vi "AlliGator All ROIs Decay Fit.vi"(8 "error in (no error)":errorcluster, 10 "Lifetime Graph":refnum<vi>, 11 "AlliGator Internal Variables DVR":refnum<data-value>) -> (0 "error out":errorcluster, 1 "Message":string, 3 "AlliGator Internal Variables DVR":refnum<data-value>)   [LabVIEW 2021, in "AlliGator Decay Fit.lvlib"]
doc: "Fits all ROI decays with the selected model, using a common IRF for all ROIs."
uses:
  AlliGator Decay Fit.lvlib
  Internal Variables/AlliGator Internal Variables v2.ctl
  <vilib>/vision/Image Controls.llb/IMAQ Image.ctl
  Internal Variables/AlliGator Gate Image Set.ctl
  Files/AlliGator FLI Dataset Type.ctl
  Files/AlliGator Data Series Type.ctl
  Dual-Channel Datasets/AlliGator Dataset Channel.ctl
  Settings/AlliGator Gate Arithmetic.ctl
  Source Image/AlliGator Displayed Image.ctl
  Image/Named ROI Description.ctl
  Phasor Graph/AlliGator Decay Metadata v3.ctl
  Decay Preprocessing/AlliGator Decay Background Subtraction Info.ctl
  Decay Preprocessing/AlliGator Baseline Subtraction Method.ctl
  Graphs/XY Graph/XY Graph Plot Shift Parameters.ctl
  Graphs/XY Graph/XY Graph Plot Shift Method.ctl
  Decay Preprocessing/AlliGator Decay Extrapolation Parameters.ctl
  Phasor/Calibration Phasor (m, phi).ctl
  Phasor/Phasor Reference Series.ctl
  Phasor/Phasor Calibration Map v2.ctl
  Phasor/Phasor (g, s).ctl
  Phasor Graph/AlliGator Raw Phasor Plot Data v5.ctl
  Phasor/Phasor Standard Deviation Options.ctl
  Phasor Plot/AlliGator Phasor Multi-Harmonic Data.ctl
  Phasor/Phasor Harmonic Data.ctl
  Decay Fit Parameter Map/AlliGator Decay Fit Options & Parameters v4.ctl
  Fits/IRF(X)PSED/Decay Fit Options v4.ctl
  Fits/Decay Convolution/Decay Model.ctl
  Fits/Residual Type.ctl
  Fits/IRF(X)PSED/Fit Weights Type v2.ctl
  Fits/Non-linear Fitting Method v2.ctl
  Fits/Fit Calculation Method.ctl
  Fits/Non-linear Fitting Algorithm.ctl
  AlliGator Decay Fit Parameter Constraints 2.ctl
  Fits/IRF(X)PSED/Decay Fit Parameters In List.ctl
  Fits/IRF(X)PSED/MLE Baseline Offset Type.ctl
  Decay Preprocessing/AlliGator Decay Preprocessing Parameters.ctl
  Fits/IRF(X)PSED/Decay Fit Parameters & Derived Quantities List v2.ctl
  Fits/IRF(X)PSED/Decay Fit Result Constraint.ctl
  Decay Fit Parameter Map/AlliGator Parameter Maps Data.ctl
  Globals, Variables, Constants/AlliGator Variables List.ctl
  Settings/AlliGator Settings List.ctl
  Rich Text Box/Text Format List.ctl
  Graphs/XY Graph/XY Graph Selected Plot Info+Flag.ctl
  Graphs/XY Graph/XY Graph Refnum.ctl
  <vilib>/Utility/miscctls.llb/LVPoint32TypeDef.ctl
  Variant/Variant to Data/Variant to U16.vi
  Variant/Variant to Data/Variant to Boolean.vi
  Globals, Variables, Constants/AlliGator Abort.vi
  <vilib>/Utility/error.llb/Error Cluster From Error Code.vi
  <vilib>/ErrorRing/Error Ring.xnode
  Globals, Variables, Constants/AlliGator Globals, Variables & Constants.lvlib
  Image/Image.lvlib
  Decay Processing/AlliGator Decay Processing.lvlib
  Source Image/AlliGator Source Image.lvlib
  Strings/Strings.lvlib
  Time/Time.lvlib
  Graphs/XY Graph/XY Graph Add-Ons.lvlib
  Settings/AlliGator Settings.lvlib
  Decay Preprocessing/AlliGator Decay Preprocessing.lvlib
  Fits/Fits.lvlib
  Variant/Variant to Data/Variant to Data.lvlib
  Notebook/Notebook.lvlib
  GUI/GUI.lvlib
  Utilities/Utilities.lvlib
  Error/Error.lvlib
  Decay Fit Parameter Map/AlliGator Decay Fit Parameter Map.lvlib
  Phasor/Phasor.lvlib
  Files/AlliGator Files.lvlib
  Internal Variables/AlliGator Internal Variables.lvlib
  Phasor Graph/AlliGator Phasor Graph.lvlib
  Phasor Plot/AlliGator Phasor Plot.lvlib
  Dual-Channel Datasets/AlliGator Dual-Channel Datasets.lvlib
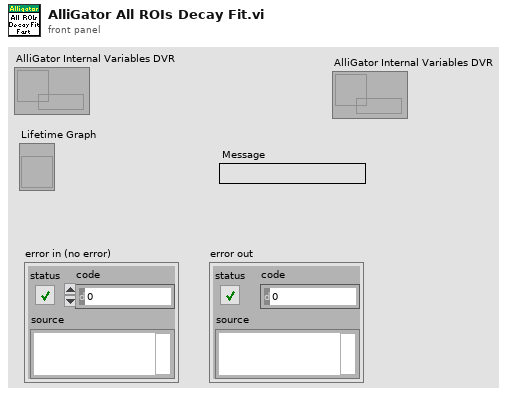
[diagram p1: front panel]
types:
  T1 = typedef "AlliGator Decay Fit.lvlib/AlliGator Decay Fit Output Options.ctl" = cluster{"Fit Model":T2, "Decay Fit Parameter Array":T3[]}
  T2 = typedef "Fits.lvlib/Decay Model.ctl" = enum16{"1-Exponential", "2-Exponentials"}
  T3 = typedef "Fits.lvlib/Decay Fit Parameters & Derived Quantities List v2.ctl" = enum16{"Offset", "Baseline", "A_1", "tau_1", "A_2", "tau_2", "<tau>_a", "f1_a", "f2_a", "<tau>_i", "f1_i", "f2_i", "-", "R^2", "Chi^2"}
  T4 = typedef "AlliGator Globals, Variables & Constants.lvlib/AlliGator Variables List.ctl" = enum16{"---- GUI ----", "GUI:Initialization Status", "GUI:State Indicators Refnum", "GUI:Original AlliGator Menu Items", "GUI:Current Action Loop State", "GUI:Script in progress", "GUI:Playback", "GUI:Loop Playback", "GUI:Search ROI Used", "GUI:Search ROI", "Decay Graph Max Legend Size", "Intensity Graph Max Legend Size", "Decay Statistics Graph Max Legend Size", "Phasor Graph Max Legend Size", "Phasor Ratio Graph Max Legend Size", "Lifetime Graph Max Legend Size", "---- Files ----", "Files:Export Dataset Frames as Individual Files", "Files:Show Batch Export Help Balloons", "Files:Frames in Dataset", "Files:ptu File Frame Start Indices", "Files:Current Frame in Dataset", "Files:Current Frame Timestamp", "Files:Dataset Loaded", "Files:Dataset Metadata", "Files:Dataset Channel", "Files:Dataset Data Description", "Files:Background Dataset Metadata", "Files:Background Dataset Channel", "Files:Background Dataset Data Description", "Files:Background File Subtraction", "Files:Background File Path", "Files:Background File Pile-up Correction", "Files:Background File Pixel Well Capacity", "Files:Background File Scaling Factor", "Files:Current Dataset Load Settings", "Files:Dataset Path", "Files:ICCD-specific Information", "Files:Macrotime Gate Separation", "------ Python Plugins ------", "Python Plugins:Information", "Python Plugins:Python Session", "Python Plugins:Valid Python Session?", "---- Source Image ----", "Source Image:ROIs", "Source Image:Current ROI", "Source Image:ROI Event Refnum", "X_Source Image:Display Range", "X_Source Image:Palette Information", "X_Source Image:Type of Displayed Image", "X_Time Gate Slider", "Source Image:Palette List", "Source Image:Scale", "Source Image:ROI Overlay Color", "Source Image:Overlay to Erase", "Source Image:Is Displayed Image Accumulated", "Source Image:White Light Image Modified", "Source Image:Mask Image Modified", "---- Image Profile Window ----", "Image Profile:Window Event Refnum", "Image Profile:IntensityType", "Image Profile:Intensity Average Type", "Image Profile:Intensity-weighted SDV", "Image Profile:Box Profile Type", "Image Profile:Window Open", "Image Profile:Plotted Fit Parameter", "------ Phasor Graph -------", "Phasor Graph:Show Line", "---- Phasor Plot ---", "Phasor Plot:Parameters Changed", "Phasor Plot:FLI Dataset Modified since last Calculation", "Phasor Harmonics Data", "Selected Phasor Harmonics", "Phasor Harmonic Manager Event Refnum", "Phasor Plot:ROIs", "Phasor Plot:Current ROI", "Phasor Plot:ROI Event Refnum", "Phasor Plot:Image Reference Points", "Phasor Plot:Computed", "Phasor Plot:Palette Information", "Phasor Plot:Palette List", "Phasor Plot:Phasor Ratio Palette Information", "Phasor Plot:Phasor Ratio Palette List", "Phasor Plot:Image Scale", "Phasor Plot:Image Overlay to Erase", "Phasor Plot:Image Elements to Update", "Phasor Plot:Current Calculation Parameters", "Phasor Plot:Current Calibration Options", "Phasor Plot:Reset Cumulated Phasor Plot", "Phasor Plot:Reference 1", "Phasor Plot:Lifetime Reference 1", "Phasor Plot:Reference 1 Frequency", "Phasor Plot:Reference 2", "Phasor Plot:Lifetime Reference 2", "Phasor Plot:Reference 2 Frequency", "---- Decay Analysis ----", "Number of Selected Decays to Fit", "LS Fit Results", "LAR Fit Results", "BS Fit Results", "Last Decay Max - Min", "Best Fit Parameters", "Best Fit Parameter Names", "Actual Size X", "Actual Size Y", "Binning X", "Binning Y", "Actual # Gates", "Dataset Number", "Gates to...", "Gates Skipped", "Gates to keep", "Gate Step", "Gate Separation", "Reversed Gates", "Pile-up Correction", "Pixel Well Capacity", "Background Subtracted", "Background Subtraction Method", "Background Definition Range", "Background File (deprecated)", "Number of Dataset Accumulated", "Array of Accumulated Dataset Paths", "Do Averaged Datasets", "Destination File Path", "Process Plot Target", "Use 1/D as Phasor Frequency", "---- Decay Fit Parameter Map -----", "Decay Fit Parameter Map:Palette Information", "Decay Fit Parameter Map:Palette List", "Decay Fit Parameter Map:X Resolution", "Decay Fit Parameter Map:Y Resolution", "Decay Fit Parameter Map:Use Decay Fit Result Constraints", "Decay Fit Parameter Map:Decay Fit Result Constraints", "Decay Fit Parameter Map:Decay Fit Result Constraints Applied", "---- Parameter Map ----", "Parameter Map:Palette Information", "Parameter Map:Palette List", "------- Local Decay Window ---------", "Local Decay Graph Window:Event Refnum", "Local Decay Graph Window:Use normalized IRF for convolution", "----- Miscellaneous ----", "Misc:Skippable Dialog Windows Status"}
  T5 = typedef "IMAQ Image.ctl" = refnum<image>
  T6 = typedef "AlliGator Settings.lvlib/AlliGator Settings List.ctl" = enum16{"GUI:Visible Settings Tab", "GUI:Last Run Version", "Source Image:Use Image Histogram for Contrast", "Source Image:Low Count Pixels Rejection Options", "Source Image:High Count Pixels Rejection Options", "Source Image:Use Image Brightness", "Source Image:Blend Overlay with Image Background", "Source Image:Use Fixed ROI Diameter", "Source Image:ROI Diameter", "Source Image:ROI Center Color", "Source Image:Peak Threshold", "Source Image:Intensity Threshold", "Source Image:Image Binning Options", "Source Image:Image Smoothing Options", "Source Image:Image Histogram Active", "Source Image:Invert Binary Mask", "Source Image:Hot Pixel Removal", "Source Image:Overlay Analyzed ROI Center", "Source Image:Auto-Adjust Contrast", "Source Image:Histogram Lower Percentile", "Source Image:Histogram Upper Percentile", "Source Image:Save Source Image", "Source Image:Scale Bar Options", "Source Image:Image Resolution (Pixel Size)", "Source Image:Flatfield Correction", "Source Image:Show Dead Left Columns Correction", "Source Image:Dead Left Columns Correction", "Source Image:Image Pre-Processing Operations Order", "Source Image:Overlay ROI Median", "Source Image:Median Overlay Color", "Data Information:Gate Width", "Data Information:Nanotime Gate Separation", "Data Information:Macrotime Gate Separation", "Data Information:Gate Step", "Data Information:# Gates", "Data Information:Gate Image Exposure", "Data Information:Gate Image Integration", "Data Information:Gates to Skip", "Data Information:Gates to Keep", "Data Information:Define Gates to", "Data Information:Channel Name", "Data Information:Available Channel Names", "Data Information:Channel Arithmetic", "Data Information:Background File Subtraction", "Data Information:Background File", "Data Information:Background Scaling Factor", "Data Information:Background Pile-up Correction", "Data Information:Background Pixel Well Capacity", "Data Information:Laser Period", "Data Information:SYNC Period", "Data Information:Pile-up Correction", "Data Information:Pixel Well Capacity", "Data Information:Dataset Scaling Factor", "Fluorescence Decay_Decay Pre-Processing:Reverse Gates", "Fluorescence Decay_Decay Pre-Processing:Verbose Decay Pre-Processing", "Fluorescence Decay_Decay Pre-Processing:Use Decay Pre-Processing", "Fluorescence Decay_Decay Pre-Processing:Background Subtraction", "Fluorescence Decay_Decay Pre-Processing:Background Definition Range", "Fluorescence Decay_Decay Pre-Processing:Baseline Subtraction Method", "Fluorescence Decay_Decay Pre-Processing:Decay Pre-Processing Operations Order", "Fluorescence Decay_Decay Pre-Processing:Smoothing Parameter", "Fluorescence Decay_Decay Pre-Processing:Shift Decay", "Fluorescence Decay_Decay Pre-Processing:Decay Shift Parameters", "Fluorescence Decay_Decay Pre-Processing:Fold Decay", "Fluorescence Decay_Decay Pre-Processing:# Folds", "Fluorescence Decay_Decay Pre-Processing:1-Normalize Decay", "Fluorescence Decay_Decay Pre-Processing:[0-1]-Normalize Decay", "Fluorescence Decay_Decay Pre-Processing:Smoothen Decay", "Fluorescence Decay_Decay Pre-Processing:Extrapolate Decay", "Fluorescence Decay_Decay Pre-Processing:Use Periodicity", "Fluorescence Decay_Decay Pre-Processing:Use Cursors", "Fluorescence Decay_Decay Pre-Processing:Tail Fraction", "Fluorescence Decay_Decay Pre-Processing:Head Fraction", "Fluorescence Decay_Decay Pre-Processing:Additional Points", "Fluorescence Decay_Decay Pre-Processing:Straighten Decay", "Fluorescence Decay_Decay Pre-Processing:Constant Background", "Fluorescence Decay_Decay Pre-Processing:Pixel-Normalize Decay", "Fluorescence Decay_Advanced Analysis:Extract IRF instead of Decay", "Fluorescence Decay_Advanced Analysis:IRF Extraction Options", "Fluorescence Decay_Advanced Analysis:IRF Optimization Options", "Fluorescence Decay_Advanced Analysis:Square Pulse Options", "Fluorescence Decay_Advanced Analysis:IRF Order", "Fluorescence Decay_Advanced Analysis:IRF Time Constants", "Fluorescence Decay_Advanced Analysis:Wavelet Analysis Options", "Fluorescence Decay_Advanced Analysis:Average Lifetime Options", "Fluorescence Decay_Fit Options:Fit Options", "Fluorescence Decay_Fit Options:Use Legacy Fitting Approach", "Fluorescence Decay_Fit Options:Use Data Information Laser Period", "Fluorescence Decay_Fit Parameters:Displayed Fit Parameters", "Fluorescence Decay_Fit Parameters:Fit Parameter Constraints", "Fluorescence Decay_Fit Parameters:Export Tabulated Results", "Fluorescence Decay_Fit Parameters:MLE Baseline Offset Type", "Fluorescence Decay_Fit Parameters:MLE Baseline Offset", "Fluorescence Decay_Fit Parameters:Guess Parameter Names", "Fluorescence Decay_Fit Parameters:Guess Parameter Values", "Fluorescence Decay_Fit Parameters:Guess Parameters Options", "Fluorescence Decay_Fit Parameters:Optimal Offset Selection Criterion", "Fluorescence Decay_Styles:Show Last Decay Only", "Fluorescence Decay_Styles:Decay Graph Color Array", "Fluorescence Decay:Decay Graph Active", "Fluorescence Decay Statistics:Min Peak Value", "Fluorescence Decay Statistics:Reject Low Decay Peak Pixels", "Fluorescence Decay Statistics:Reject High Decay Peak Pixels", "Fluorescence Decay Statistics:Max Peak Value", "Time Traces:Use File Timestamp", "Time Traces:Time Step", "Time Traces:Use Intensity Correction File", "Time Traces:Intensity Correction File", "Phasor Plot:Phasor Plot Smoothing Options", "Phasor Plot:Phasor Plot Size", "Phasor Plot:Phasor Plot Graphics Options", "Phasor Plot:Cumulative Phasor Plot", "Phasor Plot:Use Phasor Brightness", "Phasor Plot:Blend Overlay with Phasor Background", "Phasor Plot:Save Phasor Plot", "Phasor Plot:Show References", "Phasor Plot:Phasor Ratio Decay Range", "Phasor Plot:Exponential Fading", "Phasor Plot:Phasor Ratio Reference Colors", "Phasor Plot:Reference Radius", "Phasor Plot:Show Color Map Vertices", "Phasor Plot:Phasor Plot Active", "Phasor Plot:Phasor Ratio Color Map Type", "Phasor Plot:Phasor Ratio Color Map", "Phasor Plot:Phasor Ratio Display Range", "Phasor Plot:Selected Image ROI(s)", "Phasor Plot:All Image ROIs", "Phasor Plot:Selected Phasor Plot ROI(s)", "Phasor Plot:All Phasor Plot ROIs", "Phasor Plot:Phasor Ratio Color-Coded Quantity", "Phasor Plot:Store Phasor Harmonics", "Phasor Plot:Draw Reference Segment", "Phasor Plot:User-Defined Quantity", "Phasor Plot:Color Scale High Color", "Phasor Plot:Color Scale Low Color", "Phasor Plot:Intensity-weighted Phasor Plot", "Phasor Graph:Phasor Frequency", "Phasor Graph:Phasor Ratio Type", "Phasor Graph:Pixel-level Phasor Computation", "Phasor Graph:Save Phasor Graph", "Phasor Graph:Phasor Graph Active", "Phasor Graph:Phasor SDV Options", "Phasor Graph:Intensity-weighted Phasor Graph", "Phasor Graph:Define Shortest Lifetime as", "Phasor Calibration:Use Backup Calibration if needed", "Phasor Calibration:Backup Calibration Type", "Phasor Calibration:Calibration Type", "Phasor Calibration:Calibration Lifetime", "Phasor Calibration:Calibration Map Algorithm", "Single-Exponential Phasor Locus (SEPL):Gate Parameters", "Single-Exponential Phasor Locus (SEPL):User-defined Gate", "Single-Exponential Phasor Locus (SEPL):User-defined IRF", "Single-Exponential Phasor Locus (SEPL):Phasor Parameters", "Single-Exponential Phasor Locus (SEPL):Decay & IRF Parameters", "Single-Exponential Phasor Locus (SEPL):Display Parameters", "Lifetime Analysis:Decay Analysis Parameters", "Lifetime Analysis:Lifetime Map Active", "Plugins:Python Settings", "Miscellaneous:Verbose Mode", "Miscellaneous:Beep after Script", "Miscellaneous:Saved Image File Format", "Miscellaneous:Exported Gate Image Settings", "Miscellaneous:Include Loading in Timing", "Miscellaneous:Verbose Settings Mode", "Miscellaneous:Histogram Options", "Miscellaneous:Beep on Error", "Miscellaneous:# Logical Processors Used", "Miscellaneous:ROI Description Max Characters", "Miscellaneous:Verbose Error Mode", "Miscellaneous:Transparent Mask Color"}
  T7 = typedef "Image.lvlib/Named ROI Description.ctl" = cluster{"ROI Descriptor":T8, "ROI Name":string, "Overlay Color":u32}
  T8 = typedef "ROI Descriptor" = cluster{"Global Rectangle":i32[], "Contours":cluster{"ID":enum32{"External", "Internal"}, "Type":u32, "Coordinates":i32[]}[]}
  T9 = typedef "Notebook.lvlib/Text Format List.ctl" = enum16{"Message", "Result", "Error", "Setting", "Verbose", "Warning"}
  T10 = typedef "XY Graph Add-Ons.lvlib/XY Graph Selected Plot Info+Flag.ctl" = cluster{"Multiplot XY Graph":T11, "Mouse Coordinates":T12, "Plot Index":i32, "Flag":bool}
  T11 = typedef "XY Graph Add-Ons.lvlib/XY Graph Refnum.ctl" = refnum<vi>
  T12 = typedef "LVPoint32TypeDef.ctl" = cluster{"Horizontal":i32, "Vertical":i32}
  T13 = typedef "AlliGator Internal Variables.lvlib/AlliGator Internal Variables v2.ctl" = cluster{"----------------------------- Images -----------------------------":u8, "Displayed Image":T5, "White Light Image":T5, "Mask Image":T5, "ROI Mask Image":T5, "Current Dataset Images 1":T14, "Background Dataset Images 1":T14, "Current Dataset Images 2":T14, "Background Dataset Images 2":T14, "Current Dataset Arithmetic Images":T14, "Accumulated Dataset Images 1":T14, "Accumulated Dataset Images 2":T14, "Accumulated Dataset Arithmetic Images":T14, "----------------------------- File Paths -----------------------------":u8, "Phasor Plot Image":T5, "Decay Fit Parameter Map Image":T5, "Parameter Map Image":T5, "Single Data Point Path":path, "White Light Image Path":path, "Mask Image Path":path, "Time-Series Folder":path, "[Time-Series Paths]":path[], "----------------------------- FLI Dataset -----------------------------":u8, "Current Dataset":i32, "Single Dataset Type":T15, "Current Folder":string, "AlliGator Data Series Type":T16, "# Datasets":i32, "Dual-Channel Dataset":bool, "Selected Channel Name":string, "Dataset Channel":T17, "Channel Arithmetic":T18, "Dual-Channel Background Dataset":bool, "Background Channel":T17, "Dual-Channel Accumulated Dataset":bool, "Start Time":dbl, "[Time-Series Timestamps]":dbl[], "[Intensity Corrections]":dbl[], "Time Series Script":bool, "Type of Displayed Image":T19, "Gate Image Slide":u16, "# Gates":i32, "ROIs":T7[], "----------------------------- Decays -----------------------------":u8, "ROI Decay":cluster{"t Array":dbl[], "I Array":dbl[]}, "Valid Decay":bool, "Decay  Metadata":T20, "Reference Decay Plot Name":string, "Reference Decay":cluster{"t Array":dbl[], "I Array":dbl[]}, "Decay Shift Plot":cluster{"Time Stamps":dbl[], "Decay Shifts":dbl[]}, "[Decays Max Values]":sgl[], "[Decays Min Values]":sgl[], "----------------------------- Calibration -----------------------------":u8, "Calibration Phasor":T26, "Calibration Phasor Series":T27, "Phasor Calibration Map":T28, "Calibration Map MD5 Digest":string, "----------------------------- Phasor Graph -----------------------------":u8, "Last Raw Phasor":T29, "Last Calibrated Phasor":T29, "Last Calibrated Phasor SDV":T29, "Phasor Graph:Phasor Plot":cluster{"g Array":dbl[], "s Array":dbl[]}, "Phasor Graph:Phasor SDV Plot":cluster{"g Array":dbl[], "s Array":dbl[]}, "[Phasor Graph:Raw Phasor Plots]":T30[], "Phasor Plot locked to Ref 1":i32, "[Phasor Plot(s) locked to Ref 1]":i32[], "[Phasor Plot(s) locked to Ref 2]":i32[], "[Pixel Phasors]":T29[], "----------------------------- Phasor Plot -----------------------------":u8, "[[Sum Image]]":dbl[][], "[[CSG Phasors]]":csg[][], "[[Valid Pixel?]]":bool[][], "[[Phasor Ratios]]":dbl[][], "[[Average Lifetimes]]":dbl[][], "Amplitude Weighted Average Lifetime":bool, "I/m/phi Dataset":cluster{"I/m/phi Dataset?":bool, "Base Frequency":dbl[unit], "Harmonic Orders":u8[]}, "Multi Phasor Plot Data":T32, "----------------------------- Decay Fit Parameter Map -----------------------------":u8, "Decay Fit Options & Parameters":T34, "Fit Options: Decay Preprocessing Parameters":T44, "Fit Options: Reference Decay":cluster{"t Array":dbl[], "I Array":dbl[]}, "Is Full Image Parameters Map":bool, "Is Single-Pixels Parameters Map":bool, "NLSF Parameters Map X Resolution":i32, "NLSF Parameters Map Y Resolution":i32, "[Single Decay Fit Parameters]":dbl[], "Fit Model":T2, "[[Multiple Decays Fit Parameters]]":dbl[][], "[[Multiple Decays Fit Parameter SDVs]]":dbl[][], "[[IRFs]]":dbl[][], "[ROI Descriptors]":T8[], "IRF Array Time Axis":dbl[], "Decay Array Time Axis":dbl[], "[Decay Fit Parameter Names]":T3[], "[Decay Sum]":dbl[], "Array of Decay Fit Result Constraints":T45[], "Selected ROIs Array":bool[], "----------------------------- Parameter Maps -----------------------------":u8, "[Map Set Names]":string[], "[Parameter Maps]":T46[], "[[User-defined Quantities]]":dbl[][], "User-defined Quantity":string}
  T14 = typedef "AlliGator Internal Variables.lvlib/AlliGator Gate Image Set.ctl" = cluster{"SGL Gate Images":T5[], "SGL Sum Image":T5, "SGL Max Image":T5, "SGL Min Image":T5}
  T15 = typedef "AlliGator Files.lvlib/AlliGator FLI Dataset Type.ctl" = enum16{"HDF5 FLI Dataset", "Gate Image Folder", ".sdt FLI Dataset (Becker & Hickl)", ".ptu FLI Dataset (PicoQuant)", "SS1 FLI Dataset", "SS2 FLI Dataset", "I/m/phi Dataset", ".bin FLI Dataset (PicoQuant Binned)", ".bin FLI Dataset (Piccolo Binned)", ".mat FLI Dataset"}
  T16 = typedef "AlliGator Files.lvlib/AlliGator Data Series Type.ctl" = enum16{"Not a Supported Series", "Gate Images Folder Series", "SwissSPAD 2 Dataset Series", "B&H FLI Dataset Series", "PicoQuant PTU FLI Dataset Series", "PicoQuant BIN FLI Dataset Series", "Piccolo hist BIN FLI Dataset Series", "HDF5 FLI Dataset Series"}
  T17 = typedef "AlliGator Dual-Channel Datasets.lvlib/AlliGator Dataset Channel.ctl" = enum16{"G2", "INT"}
  T18 = typedef "AlliGator Settings.lvlib/AlliGator Gate Arithmetic.ctl" = enum16{"None", "INT-G2", "G2/INT*<INT>", "(1 - G2/INT)*<INT>"}
  T19 = typedef "AlliGator Source Image.lvlib/AlliGator Displayed Image.ctl" = enum16{"Single Gate", "Sum of All Gates", "Max of All Gates", "Min of All Gates", "-", "White Ligth Image", "Mask Image"}
  T20 = typedef "AlliGator Phasor Graph.lvlib/AlliGator Decay Metadata v3.ctl" = cluster{"ROI Descriptor":T8, "ROI Center":cluster{"X":i32, "Y":i32}, "Decay Background Subtraction Info":T21, "Decay Reverted":bool, "Decay Smoothened":bool, "Decay Straightened":bool, "Fitted Tau (Decay Straightening)":dbl, "Decay Shift Parameters":T23, "Decay Shifted":bool, "Decay Extrapolated":bool, "Decay Extrapolation Parameters":T25, "Decay Normalized":bool, "Fold Decay":bool, "# Folds":u32}
  T21 = typedef "AlliGator Decay Preprocessing.lvlib/AlliGator Decay Background Subtraction Info.ctl" = cluster{"Laser Period":dbl[unit], "Gate Duration":dbl[unit], "Baseline Subtraction Method":T22, "Background Definition Range":cluster{"Min Gate":dbl[unit], "Max Gate":dbl[unit]}, "Total Intensity w/o Bkgd Subtraction":dbl, "Bkgd-subtracted Intensity (exp)":dbl, "# Data Points":i32, "Background/Gate":dbl, "Fitted Lifetime":dbl[unit], "Bkgd-subtracted Intensity (theo)":dbl}
  T22 = typedef "AlliGator Decay Preprocessing.lvlib/AlliGator Baseline Subtraction Method.ctl" = enum16{"Mean", "Min", "Square Gated Single-Exponential", "File", "Constant"}
  T23 = typedef "XY Graph Add-Ons.lvlib/XY Graph Plot Shift Parameters.ctl" = cluster{"Type":T24, "Shift":dbl[unit], "Threshold":dbl, "Rotate":bool}
  T24 = typedef "XY Graph Add-Ons.lvlib/XY Graph Plot Shift Method.ctl" = enum16{"Default", "CFD", "Threshold", "Cross-Correlation"}
  T25 = typedef "AlliGator Decay Preprocessing.lvlib/AlliGator Decay Extrapolation Parameters.ctl" = cluster{"Additional Points":u32, "Head Fraction":dbl, "Fitted Tau":dbl, "Use Periodicity":bool, "Use Cursors":bool, "Tail Fraction":dbl}
  T26 = typedef "Phasor.lvlib/Calibration Phasor (m, phi).ctl" = cluster{"m":dbl, "phi":dbl, "Phasor Frequency":dbl[unit], "Reference Lifetime":dbl[unit]}
  T27 = typedef "Phasor.lvlib/Phasor Reference Series.ctl" = cluster{"m Array":dbl[], "phi Array":dbl[], "Phasor Frequency":dbl[unit], "Calibration Lifetime":dbl[unit]}
  T28 = typedef "Phasor.lvlib/Phasor Calibration Map v2.ctl" = cluster{"Phasor Frequency":dbl[unit], "Calibration Lifetime":dbl[unit], "ROI Centers":cluster{"X":i32, "Y":i32}[], "ROI Descriptors":T8[], "Map Resolution X":i32, "Map Resolution Y":i32, "z Array":cdb[]}
  T29 = typedef "Phasor.lvlib/Phasor (g, s).ctl" = cluster{"g":dbl, "s":dbl}
  T30 = typedef "AlliGator Phasor Graph.lvlib/AlliGator Raw Phasor Plot Data v5.ctl" = cluster{"Phasor Plot Name":string, "Raw Phasor Plot":T29[], "Phasor Frequency":dbl[unit], "[Decay Metadata]":T20[], "Raw Phasor Plot SDV":T29[], "Phasor SDV Options":T31, "[Calibration Phasor]":T26[], "Intensity Array":dbl[]}
  T31 = typedef "Phasor.lvlib/Phasor Standard Deviation Options.ctl" = cluster{"Compute Estimated SDV":bool, "# Replicas":u32, "Use Estimated Average Phasor":bool}
  T32 = typedef "AlliGator Phasor Plot.lvlib/AlliGator Phasor Multi-Harmonic Data.ctl" = cluster{"Base Frequency":dbl[unit], "# Harmonics":u8, "Harmonic Orders":u8[], "Phasor Plot Settings Checksum":u64, "Phasor Harmonic Data Array":T33[]}
  T33 = typedef "Phasor.lvlib/Phasor Harmonic Data.ctl" = cluster{"Phasor Harmonic Name":string, "Phasor Plot Settings Checksum":u64, "Phasor Frequency":dbl[unit], "Base Frequency":dbl[unit], "Harmonic Order":u8, "Phasor Plot Parameters":string, "Phasor Array [[CSG]]":csg[][], "Dataset File Path":path}
  T34 = typedef "AlliGator Decay Fit Parameter Map.lvlib/AlliGator Decay Fit Options & Parameters v4.ctl" = cluster{"SYNC Period":dbl[unit], "Fit Options":T35, "Fit Parameter Constraints":T41[], "MLE Baseline Offset":dbl, "MLE Baseline Offset Type":T43}
  T35 = typedef "Fits.lvlib/Decay Fit Options v4.ctl" = cluster{"Show Fit Residuals":bool, "Fit Model":T2, "Residual Type":T36, "Max Decay Percentile":dbl, "Min Decay Percentile":dbl, "Show Full Decay":bool, "Weights":T37, "Fitting Method":T38, "Compute Parameter Uncertainties":bool, "Periodic Boundaries":bool, "Model Calculation":T39, "Period":dbl[unit], "Termination Criteria":cluster{"Max Iterations":i32, "Max Function Calls":i32, "Max Time":dbl[unit], "Function Tolerance":dbl, "Parameter Tolerance":dbl, "Gradient Tolerance":dbl, "Min Lambda":dbl, "Max Lambda":dbl, "Initial Tick Count":u32}, "Offset Resolution":dbl[unit], "Use Local IRF":bool, "Fitting Algorithm":T40, "Show Confidence Interval ":bool, "Confidence Level":dbl}
  T36 = typedef "Fits.lvlib/Residual Type.ctl" = enum16{"Standard", "Normalized", "Reduced"}
  T37 = typedef "Fits.lvlib/Fit Weights Type v2.ctl" = enum16{"Unweighted", "1/Variance (Neyman)", "1/Variance (Pearson)", "Best of All"}
  T38 = typedef "Fits.lvlib/Non-linear Fitting Method v2.ctl" = enum16{"Least Square", "Least Absolute Residual", "Bisquare", "MLE", "-", "Best of All"}
  T39 = typedef "Fits.lvlib/Fit Calculation Method.ctl" = enum16{"Simulation", "Convolution", "Integration"}
  T40 = typedef "Fits.lvlib/Non-linear Fitting Algorithm.ctl" = enum16{"Levenberg-Marquardt", "Trust-Region Dogleg"}
  T41 = typedef "AlliGator Decay Fit.lvlib/AlliGator Decay Fit Parameter Constraints 2.ctl" = cluster{"Fit Parameter":T42, "Min Value":dbl, "Max Value":dbl, "Global":bool, "Used":bool}
  T42 = typedef "Fits.lvlib/Decay Fit Parameters In List.ctl" = enum16{"Offset", "Baseline", "A_1", "tau_1", "A_2", "tau_2"}
  T43 = typedef "Fits.lvlib/MLE Baseline Offset Type.ctl" = enum32{"Absolute", "Percentage"}
  T44 = typedef "AlliGator Decay Preprocessing.lvlib/AlliGator Decay Preprocessing Parameters.ctl" = cluster{"Background Subtraction":bool, "Straighten Decay":bool, "Reverse Gates":bool, "1-Normalized Decay":bool, "Smoothen Decay":bool, "Smoothing Parameter":dbl, "Shift Decay":bool, "Decay Shift Parameters":T23, "Extrapolate Decay":bool, "Additional Points":u32, "Head Fraction":dbl, "Pixel-Normalize Decay":bool, "Use Periodicity":bool, "Use Cursors":bool, "Tail Fraction":dbl, "Use Decay Pre-Processing":bool, "Fold Decay":bool, "# Folds":u32, "[0-1]-Normalized Decay":bool}
  T45 = typedef "Fits.lvlib/Decay Fit Result Constraint.ctl" = cluster{"Fit Parameter":enum16{"Offset", "Baseline", "A_1", "tau_1", "A_2", "tau_2", "<tau>_a", "f1_a", "f2_a", "<tau>_i", "f1_i", "f2_i", "-", "R^2", "Chi^2", "Max Relative Residual", "<Residual ACF>", "Residual ACF SDV", "tau_2/tau_1"}, "Min Value":dbl, "Max Value":dbl, "Use Constraint":bool}
  T46 = typedef "AlliGator Decay Fit Parameter Map.lvlib/AlliGator Parameter Maps Data.ctl" = cluster{"Map Set Name":string, "[Parameter Names]":string[], "[[Parameters]]":dbl[][], "[[Parameter SDVs]]":dbl[][], "Decay Array Time Axis":dbl[], "[[IRFs]]":dbl[][], "IRF Array Time Axis":dbl[], "X Resolution":i32, "Y Resolution":i32, "Intensity Array":dbl[]}
  T47 = typedef "AlliGator Settings.lvlib/AlliGator Pixel Counts Constraints.ctl" = cluster{"High Count Pixels Rejection Options":T48, "Low Count Pixels Rejection Options":T49}
  T48 = typedef "AlliGator Settings.lvlib/AlliGator High Count Pixels Rejection Options.ctl" = cluster{"Background High Threshold Factor":dbl, "Fixed High Background Threshold":dbl, "Reject High Count Pixels":bool, "High Percentile":dbl}
  T49 = typedef "AlliGator Settings.lvlib/AlliGator Low Count Pixels Rejection Options.ctl" = cluster{"Background Low Threshold Factor":dbl, "Fixed Low Background Threshold":dbl, "Reject Low Count Pixels":bool, "Low Percentile":dbl}
  T50 = cluster{"Decay Peak Constraint":bool, "Min":dbl, "Max":dbl}
  T51 = typedef "Rich Text Box.lvlib/Text Formatting.ctl" = cluster{"Font":string, "Text Color":T52, "Background Color":T52, "Style":T53, "Font Size":dbl, "Alignment":T54}
  T52 = typedef "Rich Text Box.lvlib/Text Colors.ctl" = enum16{"Unchanged", "Black", "Blue", "Cyan", "Maroon", "Gray", "Violet", "Green", "Light Green", "Orange", "Yellow", "Magenta", "Red", "White"}
  T53 = typedef "Rich Text Box.lvlib/Text Style.ctl" = enum16{"Regular", "Bold", "Italic", "Underline", "Strikeout"}
  T54 = typedef "Rich Text Box.lvlib/Text Alignment.ctl" = enum16{"Left", "Right", "Center"}
  T55 = cluster{"t Axis":dbl[], "ROI Intensity Array":dbl[]}
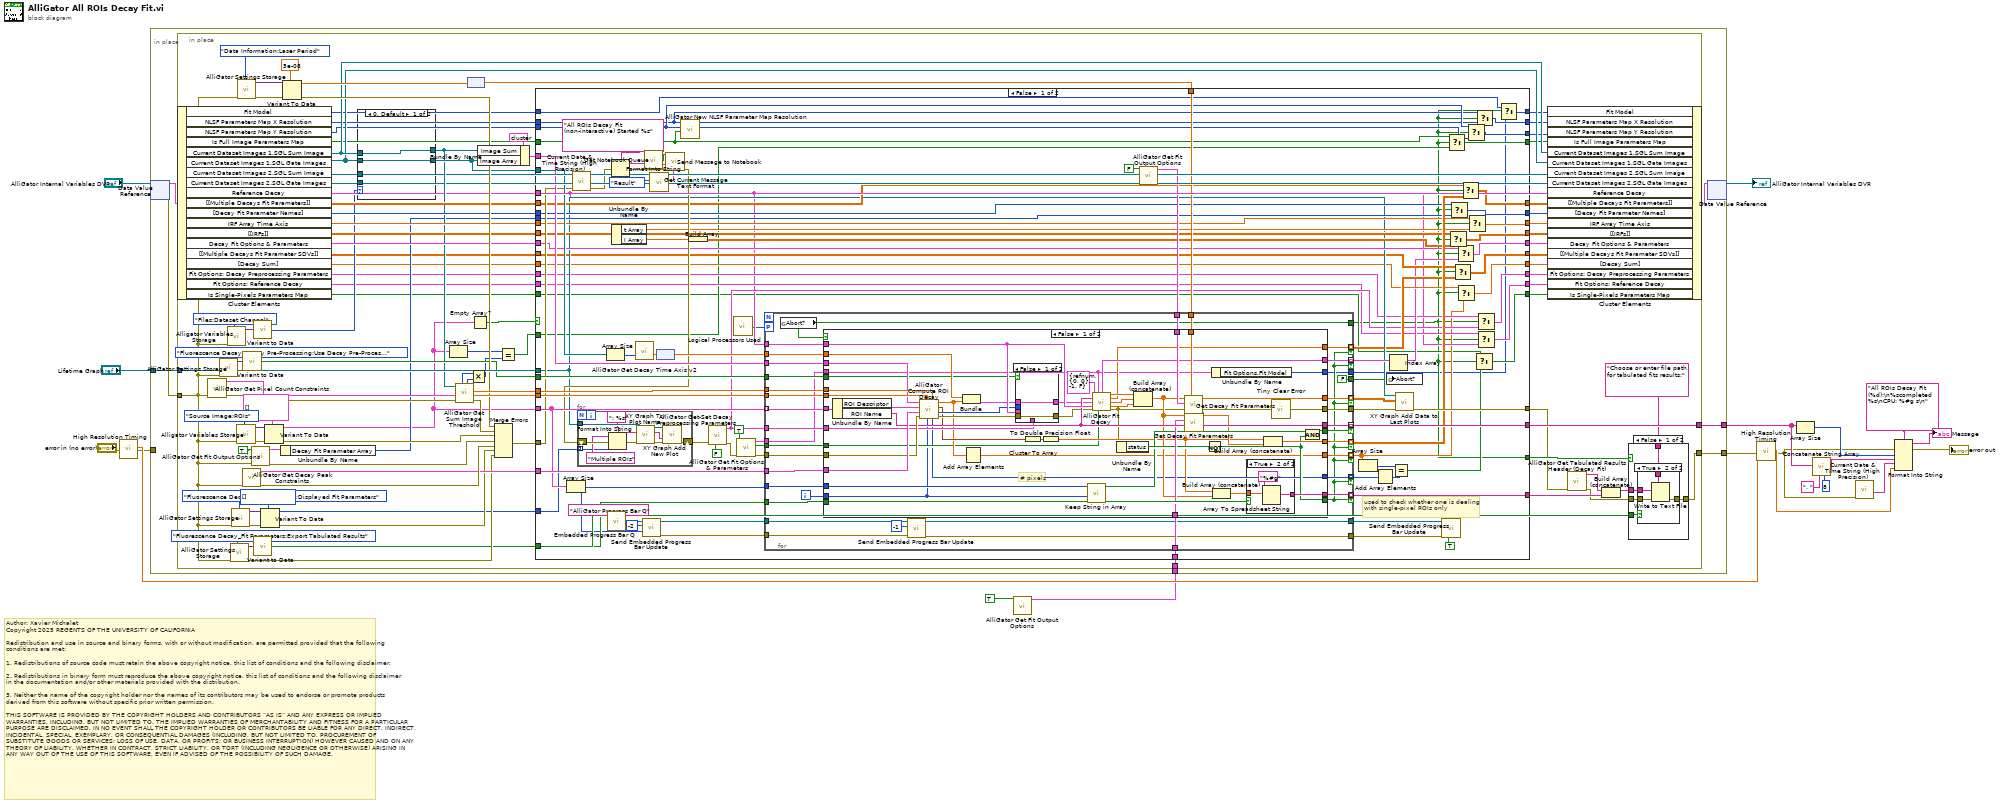
[diagram p0: block diagram]
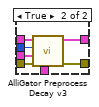
[diagram p3: hidden frame]
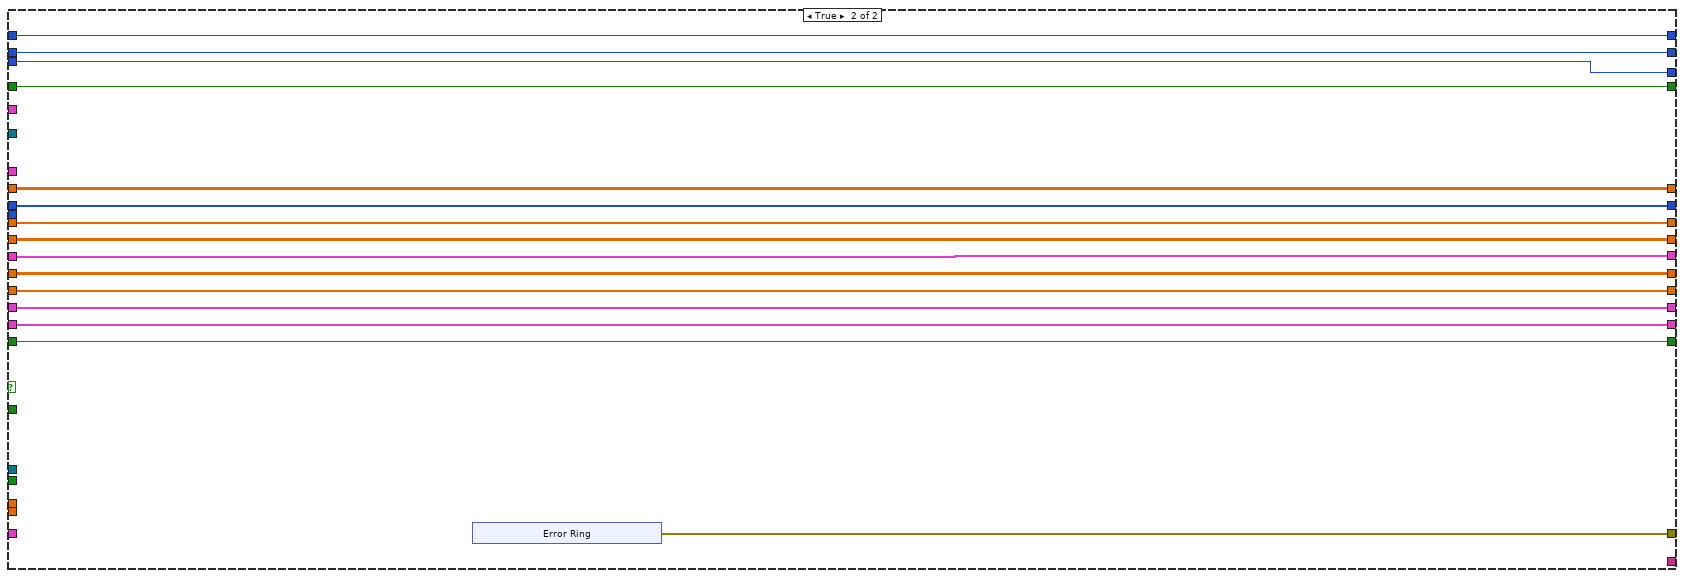
[diagram p6: hidden frame]
diagram:
  # "Author: Xavier Michalet\nCopyright 2025 REGENTS OF THE UNIVERSITY OF CALIFORNIA\n\nRedistribution and use in source and binary forms, with or without modification, are permitted provided that the following conditions are met:\n\n1. Redistributions of source code must retain the above copyright notice, this list of conditions and the following disclaimer.\n\n2. Redistributions in binary form must reproduce the above copyright notice, this list of conditions and the following disclaimer in the documentation and/or other materials provided with the distribution.\n\n3. Neither the name of the copyright holder nor the names of its contributors may be used to endorse or promote products derived from this software without specific prior written permission.\n\nTHIS SOFTWARE IS PROVIDED BY THE COPYRIGHT HOLDERS AND CONTRIBUTORS “AS IS” AND ANY EXPRESS OR IMPLIED WARRANTIES, INCLUDING, BUT NOT LIMITED TO, THE IMPLIED WARRANTIES OF MERCHANTABILITY AND FITNESS FOR A PARTICULAR PURPOSE ARE DISCLAIMED. IN NO EVENT SHALL THE COPYRIGHT HOLDER OR CONTRIBUTORS BE LIABLE FOR ANY DIRECT, INDIRECT, INCIDENTAL, SPECIAL, EXEMPLARY, OR CONSEQUENTIAL DAMAGES (INCLUDING, BUT NOT LIMITED TO, PROCUREMENT OF SUBSTITUTE GOODS OR SERVICES; LOSS OF USE, DATA, OR PROFITS; OR BUSINESS INTERRUPTION) HOWEVER CAUSED AND ON ANY THEORY OF LIABILITY, WHETHER IN CONTRACT, STRICT LIABILITY, OR TORT (INCLUDING NEGLIGENCE OR OTHERWISE) ARISING IN ANY WAY OUT OF THE USE OF THIS SOFTWARE, EVEN IF ADVISED OF THE POSSIBILITY OF SUCH DAMAGE."
  n1 = call "High Resolution Timing.vi"("Error In"="error in (no error)") -> ("elapsed (relative) seconds"=w14:dbl, "Error Out"=w9:errorcluster)  [unwired: 16 in, 1 out]
  n2 = call "AlliGator Get Fit Output Options.vi"("All Parameters?"=TRUE) -> ("Decay Fit Output Options"=w5:T1)  [unwired: 8 in, 2 out]
  n3 = in-place {
    in-place-border: [w25] -> w7
    in-place-border: [w24] -> w11
    in-place-border: w9 -> [_]
    in-place-border: "Lifetime Graph" -> [w22]
    in-place-border: w5 -> [w21]
    n4 = in-place-dvr #1("AlliGator Internal Variables DVR") -> (w27:T13, w23:errorcluster)
    n5 = in-place {
      in-place-border: w23 -> [w55]
      in-place-border: [w95] -> w25
      in-place-border: [w111] -> w24
      in-place-border: w22 -> [w103]
      in-place-border: w21 -> [w91]
      w106 = T3[] [] items=["Offset", "Baseline", "A_1", "tau_1", "A_2", "tau_2", "<tau>_a", "f1_a", "f2_a", "<tau>_i", "f1_i", "f2_i", "-", "R^2", "Chi^2"] ("Array")
      n6 = in-place-cluster #2(w27) -> ("Fit Model"=w29:T2, "NLSF Parameters Map X Resolution"=w35:i32, "NLSF Parameters Map Y Resolution"=w32:i32, "Is Full Image Parameters Map"=w43:bool, "Current Dataset Images 1.SGL Sum Image"=w49:T5, "Current Dataset Images 1.SGL Gate Images"=w48:T5[], "Current Dataset Images 2.SGL Sum Image"=w67:T5, "Current Dataset Images 2.SGL Gate Images"=w66:T5[], "Reference Decay"=w64:cluster{"t Array":dbl[], "I Array":dbl[]}, "[[Multiple Decays Fit Parameters]]"=w80:dbl[][], "[Decay Fit Parameter Names]"=w77:T3[], "IRF Array Time Axis"=w75:dbl[], "[[IRFs]]"=w74:dbl[][], "Decay Fit Options & Parameters"=w71:T34, "[[Multiple Decays Fit Parameter SDVs]]"=w52:dbl[][], "[Decay Sum]"=w51:dbl[], "Fit Options: Decay Preprocessing Parameters"=w47:T44, "Fit Options: Reference Decay"=w45:cluster{"t Array":dbl[], "I Array":dbl[]}, "Is Single-Pixels Parameters Map"=w31:bool)
      n7 = call "AlliGator Get Pixel Count Constraints.vi"("error in (no error)"=w55) -> ("error out"=w118:errorcluster, "Pixel Count Constraints"=w119:T47)  [unwired: 9 in]
      n8 = call "AlliGator Settings Storage.vi"("AlliGator Settings List"=AlliGator_Settings_List."Fluorescence Decay_Decay Pre-Processing:Use Decay Pre-Processing", "Error In"=w55) -> ("Variant Data out"=w83:variant)  [unwired: 8 in, 1 out]
      n9 = call "Alligator Variables Storage.vi"("AlliGator Variable"=AlliGator_Variables_List."Files:Dataset Channel" ("Alligator Variable"), "Error In"=w55) -> ("Data out"=w56:variant)  [unwired: 7 in, 2 out]
      n10 = call "AlliGator Settings Storage.vi"("AlliGator Settings List"=AlliGator_Settings_List."Fluorescence Decay_Fit Parameters:Export Tabulated Results", "Error In"=w55) -> ("Error Out"=w100:errorcluster, "Variant Data out"=w101:variant)  [unwired: 8 in]
      n11 = call "AlliGator Settings Storage.vi"("AlliGator Settings List"=AlliGator_Settings_List."Fluorescence Decay_Fit Parameters:Displayed Fit Parameters", "Error In"=w55) -> ("Error Out"=w108:errorcluster, "Variant Data out"=w107:variant)  [unwired: 8 in]
      n12 = call "Alligator Variables Storage.vi"("AlliGator Variable"=AlliGator_Variables_List."Source Image:ROIs" ("Alligator Variable"), "Error In"=w55) -> ("Error Out"=w121:errorcluster, "Data out"=w122:variant)  [unwired: 7 in, 1 out]
      n13 = call "AlliGator Settings Storage.vi"("AlliGator Settings List"=AlliGator_Settings_List."Data Information:Laser Period", "Error In"=w55) -> ("Error Out"=w89:errorcluster, "Variant Data out"=w90:variant)  [unwired: 8 in]
      n14 = call "AlliGator Get Decay Peak Constraints.vi"("error in (no error)"=w55) -> ("Error Out"=w114:errorcluster, "Decay Peak Constraints"=w113:T50)  [unwired: 9 in]
      n15 = call-poly "Variant to Data.vi"("Variant"=w83) -> ("Value"=w81:bool)  [unwired: 8 in]
      n16 = call "AlliGator Get Fit Output Options.vi"("Error In"=w55, "All Parameters?"=TRUE) -> ("Error Out"=w58:errorcluster, "Decay Fit Output Options"=w61:T1)  [unwired: 7 in, 1 out]
      n17 = call-poly "Variant to Data.vi"("Variant"=w56) -> ("U16 Value"=w54:u16)  [unwired: 8 in]
      n18 = call-poly "Variant to Data.vi"("Variant"=w101) -> ("Value"=w93:bool)  [unwired: 8 in]
      n19 = Variant To Data(error in=w108, type=w106, Variant=w107) -> (data=w62:T3[], error out=w104:errorcluster)
      n20 = Variant To Data(error in=w121, type=T7[] [] ("Stored ROIs in"), Variant=w122) -> (data=w41:T7[], error out=w117:errorcluster)
      n21 = Unbundle By Name(w61) -> ("Decay Fit Parameter Array"=w59:T3[])
      n22 = Variant To Data(error in=w89, type=dbl[unit] 5e-08 ("Laser Period"), Variant=w90) -> (data=w88:dbl[unit], error out=w84:errorcluster)
      n23 = case shown="0, Default" w54 {
        tunnel: [w125 w127] -> w68
        tunnel: w67 -> [_ w127]
        tunnel: w66 -> [_ w126]
        tunnel: [w124 w126] -> w69
        tunnel: w49 -> [w125 _]
        tunnel: w48 -> [w124 _]
        frame 0, Default {
        }
        frame 1 {
        }
      }
      n24 = Array Size(array=w41) -> (size(s)=w38:i32)
      n25 = call "AlliGator Get Sum Image Threshold.vi"("error in (no error)"=w118, "Pixel Counts Constraints"=w119, "Image in"=w68) -> ("error out"=w110:errorcluster, "Pixel Threshold Low"=w115:sgl, "Pixel Threshold High"=w116:sgl, "Y Resolution"=w40:i32, "X Resolution"=w39:i32)  [unwired: 2 in, 2 out]
      n26 = node(w88) -> (w85:dbl)
      n27 = Multiply(x=w39, y=w40) -> (x*y=w37:i32)
      n28 = Empty Array?(array=w41) -> (empty?=w63:bool)
      n29 = Bundle By Name(cluster=cluster{"Image Sum":T5, "Image Array":T5[]} {"Image Sum"=refnum, "Image Array"=[]} ("Images"), "Image Sum"=w68, "Image Array"=w69) -> (w112:cluster{"Image Sum":T5, "Image Array":T5[]})
      n30 = Merge Errors(w84, w110, w117, w58, w114, w104, w100) -> (w109:errorcluster)
      n31 = Equal?(x=w38, y=w37) -> (x = y?=w36:bool)
      n32 = case shown="False" w63 {
        tunnel: w116 -> [w225 _]
        tunnel: w115 -> [w224 _]
        tunnel: w113 -> [w223 _]
        tunnel: w112 -> [w222 _]
        tunnel: w69 -> [w221 _]
        tunnel: w64 -> [w156 _]
        tunnel: [w218 _] -> w111
        tunnel: w109 -> [w199 _]
        tunnel: w62 -> [w179 _]
        tunnel: w103 -> [w169 _]
        tunnel: [w216 _] -> w99
        tunnel: [w132 _] -> w96
        tunnel: [w215 w350] -> w79
        tunnel: w93 -> [w214 _]
        tunnel: [w197 w351] -> w92
        tunnel: w41 -> [w213 _]
        tunnel: w91 -> [w212 _]
        tunnel: w85 -> [w209 _]
        tunnel: w81 -> [w208 _]
        tunnel: w80 -> [w196 w351]
        tunnel: w77 -> [w195 w349]
        tunnel: [w194 w349] -> w76
        tunnel: w75 -> [w193 w348]
        tunnel: w74 -> [w192 w347]
        tunnel: [w191 w348] -> w73
        tunnel: [w190 w347] -> w72
        tunnel: w71 -> [w185 w346]
        tunnel: [w184 w346] -> w70
        tunnel: w59 -> [w171 _]
        tunnel: [w165 w345] -> w53
        tunnel: w52 -> [w164 w345]
        tunnel: w51 -> [w163 w344]
        tunnel: [w162 w344] -> w50
        tunnel: w47 -> [w160 w343]
        tunnel: [w159 w343] -> w46
        tunnel: w45 -> [w157 w342]
        tunnel: [w155 w342] -> w44
        tunnel: w43 -> [w145 w341]
        tunnel: [w149 w341] -> w42
        tunnel: w36 -> [w146 _]
        tunnel: w35 -> [w141 w340]
        tunnel: w32 -> [w143 w339]
        tunnel: [w148 w340] -> w34
        tunnel: [w147 w339] -> w33
        tunnel: w31 -> [w136 w338]
        tunnel: [w134 w338] -> w30
        tunnel: w29 -> [w133 w337]
        tunnel: [w130 w337] -> w28
        frame False {
          # "used to check whether one is dealing with single-pixel ROIs only"
          n33 = Array Size(array=w213) -> (size(s)=w176:i32)
          n34 = call "Current Date & Time String (High Precision).vi"("Error In"=w199) -> ("Error Out"=w203:errorcluster, "on <Date> at <Time>"=w182:string)  [unwired: 7 in, 2 out]
          n35 = Array Size(array=w221) -> (size(s)=w220:i32)
          n36 = call "Embedded Progress Bar Q.vi"("Progress Bar Queue Name"="AlliGator Progress Bar Q") -> ("Progress Bar Queue"=w181:refnum<queue>)  [unwired: 6 in]
          n37 = Format Into String(format string="All ROIs Decay Fit (non-interactive) Started %s", error in=w203, w182) -> (resulting string=w204:string, error out=w202:errorcluster)  [unwired: 1 in]
          n38 = Unbundle By Name(w156) -> ("t Array"=w189:dbl[], "I Array"=w188:dbl[])
          n39 = call "AlliGator Get Decay Time Axis v2.vi"("Number of Gates"=w220) -> ("t Array"=w219:dbl[unit][])  [unwired: 14 in]
          n40 = call "Send Embedded Progress Bar Update.vi"("Max Iterations N"=w176, "Current Iteration i (i or -1: standard or || iteration; 0 or -2: first standard or || iteration)"=-2 ("Current Iteration i (i or -1: standard or || iteration; 0 or -2: first standard or || iteration)"), "Progress Bar Queue in"=w181) -> ("Error Out"=w175:errorcluster, "Progress Bar Queue out"=w178:refnum<queue>)  [unwired: 7 in]
          n41 = call "Get Notebook Queue.vi"() -> ("Notebook Queue"=w201:refnum<queue>)  [unwired: 9 in]
          n42 = call "Get Current Message Text Format.vi"("Text Format"=Text_Format_List."Result") -> ("Message Formatting"=w206:T51)  [unwired: 8 in, 1 out]
          n43 = node(w219) -> (w217:dbl[])
          n44 = call "Send Message to Notebook.vi"("Text Formatting"=w206, "Error In"=w202, "Text"=w204, "Notebook Queue"=w201) -> ("Error Out"=w200:errorcluster)  [unwired: 4 in, 1 out]
          n45 = for {
            tunnel: w169 -> [w233]
            shift-right: [w235] -> w207
            shift-left: w200 -> [w231]
            tunnel: w179 -> [w227] mode=indexing
            n46 = Format Into String(format string=": %s", initial string="Multiple ROIs", error in=w231, w227) -> (resulting string=w229:string, error out=w230:errorcluster)
            n47 = call "XY Graph Try Plot Name.vi"("Error In"=w230, "Plot Name in"=w229, "XY Graph Refnum"=w233) -> ("Error Out"=w234:errorcluster, "Plot Name out"=w236:string, "XY Graph Refnum"=w226:T11)  [unwired: 5 in, 1 out]
            n48 = call "XY Graph Add New Plot.vi"("Multiplot XY Graph"=w226, "New Plot Name in"=w236, "error in (no error)"=w234) -> ("error out"=w235:errorcluster)  [unwired: 9 in, 3 out]
          }
          n49 = call "AlliGator New NLSF Parameter Map Resolution.vi"("Is Full Image Parameter Map"=w145, "Old NLSF Parameters Map Y Resolution"=w143, "Old NLSF Parameters Map X Resolution"=w141) -> (2:"New NLSF Parameters Map X Resolution"=w144:i32, 3:"New NLSF Parameters Map X Resolution"=w142:i32)  [unwired: 7 in]
          n50 = Build Array(w188) -> (w187:dbl[][])
          n51 = call "AlliGator Get-Set Decay Preprocessing Parameters.vi"("Get (F)/Set"=FALSE, "Error In"=w207) -> ("Error Out"=w154:errorcluster, "Decay Preprocessing Parameters out"=w158:T44)  [unwired: 8 in]
          n52 = call "Logical Processors Used.vi"() -> ("# Logical Processor Used"=w129:i32)  [unwired: 6 in]
          n53 = call "AlliGator Get Fit Options & Parameters.vi"("error in (no error)"=w154, "Reset Fit Options & Parameters"=TRUE) -> ("error out"=w153:errorcluster, "Use Legacy Fitting Approach"=w152:bool, "Decay Fit Options & Parameters"=w151:T34)  [unwired: 7 in]
          n54 = call "AlliGator Get Fit Output Options.vi"("All Parameters?"=FALSE) -> ("Decay Fit Output Options"=w210:T1)  [unwired: 8 in, 2 out]
          n55 = for {
            tunnel: w213 -> [w273] mode=indexing
            tunnel: w225 -> [w272]
            tunnel: w224 -> [w271]
            tunnel: w222 -> [w270]
            tunnel: w223 -> [w269]
            tunnel: w217 -> [w267]
            tunnel: w156 -> [w266]
            tunnel: [w265] -> w218 mode=indexing if=w259
            tunnel: w153 -> [w268]
            tunnel: [w264] -> w168
            tunnel: [w263] -> w216 mode=indexing if=w238
            tunnel: w214 -> [w262]
            tunnel: [w244] -> w132
            tunnel: [w258] -> w198 mode=indexing if=w238
            tunnel: w176 -> [w261]
            tunnel: w212 -> [w257]
            tunnel: w210 -> [w256]
            tunnel: w209 -> [w255]
            tunnel: w208 -> [w254]
            tunnel: [w253] -> w186 mode=indexing if=w238
            tunnel: w158 -> [w252]
            tunnel: w178 -> [w251]
            tunnel: w175 -> [w250]
            tunnel: [w249] -> w174
            tunnel: [w248] -> w173
            tunnel: [w247] -> w170 mode=indexing if=w238
            tunnel: [FALSE ("Abort?")] -> w167
            tunnel: [w243] -> w140 mode=indexing if=w238
            tunnel: [w242] -> w166 mode=indexing if=w238
            tunnel: w152 -> [w241]
            tunnel: w151 -> [w240]
            tunnel: [w239] -> w138 mode=indexing if=w238
            tunnel: [w237] -> w131
            workers-P: w129 -> [_]
            i -> [w260]
            n56 = global read "AlliGator Abort.vi" "Abort?"() -> (w244:bool)
            n57 = case shown="False" w244 {
              tunnel: w273 -> [w323 _]
              tunnel: w272 -> [w322 _]
              tunnel: w271 -> [w321 _]
              tunnel: w270 -> [w320 _]
              tunnel: w269 -> [w319 _]
              tunnel: w268 -> [w318 w336]
              tunnel: w267 -> [w317 _]
              tunnel: w266 -> [w316 _]
              tunnel: [w315 _] -> w265
              tunnel: [w314 w336] -> w264
              tunnel: [w313 _] -> w263
              tunnel: w262 -> [w312 _]
              tunnel: w261 -> [w311 _]
              tunnel: w260 -> [w274 _]
              tunnel: [w310 _] -> w259
              tunnel: [w309 _] -> w258
              tunnel: w257 -> [w308 _]
              tunnel: w256 -> [w307 _]
              tunnel: w255 -> [w306 _]
              tunnel: w254 -> [w305 _]
              tunnel: [w304 _] -> w253
              tunnel: w252 -> [w303 _]
              tunnel: [w302 _] -> w247
              tunnel: [w301 _] -> w238
              tunnel: [w280 _] -> w243
              tunnel: [w279 _] -> w242
              tunnel: w241 -> [w278 _]
              tunnel: w240 -> [w276 _]
              tunnel: [w277 _] -> w239
              tunnel: [w275 _] -> w237
              frame False {
                # "# pixels"
                n58 = Unbundle By Name(w323) -> ("ROI Descriptor"=w300:T8, "ROI Name"=w315:string)
                n59 = call "AlliGator Compute ROI Decay.vi"("Pixel Threshold High"=w322, "Loop ID"=w274, "Pixel Threshold Low"=w321, "error in (no error)"=w318, "Decay Peak  Constraints"=w319, "ROI Descriptor"=w300, "Images"=w320) -> ("error out"=w299:errorcluster, "# Valid Pixels"=w297:i32, "ROI Center"=w286:cluster{"X":i32, "Y":i32}, "Decay Points"=w281:dbl[], "# Pixels"=w277:i32)
                n60 = Bundle(w317, "Decay Points"=w281) -> (w298:cluster{dbl[], "Decay Points":dbl[]})  [unwired: 1 in]
                n61 = Add Array Elements(numeric array=w281) -> (sum=w280:dbl)
                n62 = case shown="False" w305 {
                  tunnel: w299 -> [w324 w332]
                  tunnel: w298 -> [w325 w331]
                  tunnel: w297 -> [_ w330]
                  tunnel: [w324 w329] -> w283
                  tunnel: w316 -> [_ w328]
                  tunnel: [w325 w327] -> w296
                  tunnel: w303 -> [_ w326]
                  frame False {
                  }
                  frame True {
                    n63 = call "AlliGator Preprocess Decay v3.vi"("Decay Preprocessing Parameters"=w326, "Error In"=w332, "Time-Gated Reference Decay"=w328, "# Pixels"=w330, "Decay (in)"=w331) -> ("Error Out"=w329:errorcluster, "Decay (out)"=w327:T55)  [unwired: 3 in, 2 out]
                  }
                }
                n64 = Cluster To Array(cluster=w286) -> (array=w285:i32[])
                n65 = To Double Precision Float(number=w285) -> (double precision float=w284:dbl[])
                n66 = call "Keep String in Array.vi"("Current Index"=w274, "Number of Elements"=w311) -> ("Keep String"=w289:bool)  [unwired: 9 in]
                n67 = call "AlliGator Fit Decay.vi"("Selected Plot Info + Flag"=T10 {"Multiplot XY Graph"=refnum, "Mouse Coordinates"={"Horizontal"=0, "Vertical"=0}, "Plot Index"=-1, "Flag"=FALSE}, "Decay Fit Options & Parameters"=w276, "Current Decay Name"=w315, "Current Decay"=w296, "Reference Decay"=w316, "error in (no error)"=w283, "Use Legacy Fitting Approach"=w278) -> ("Decay Fit Options & Parameters (out)"=w304:T34, "Best Fit Parameters (All)"=w294:dbl[], "Delta Best Fit Parameters (All)"=w279:dbl[], "R^2"=w293:dbl, "Reduced Chi^2"=w292:dbl, "Error Out"=w282:errorcluster)  [unwired: 3 out]
                n68 = Unbundle By Name(w282) -> ("status"=w291:bool)
                n69 = Build Array (concatenate)(w294, w293, w292) -> (w288:dbl[])
                n70 = call "Get Decay Fit Parameters.vi"("Laser Period"=w306, "Decay Fit Output Options"=w307, "Decay Fit Parameters"=w288) -> ("Displayed Decay Fits Parameters"=w302:dbl[])  [unwired: 7 in, 1 out]
                n71 = call "Get Decay Fit Parameters.vi"("Laser Period"=w306, "Decay Fit Output Options"=w308, "Decay Fit Parameters"=w288) -> ("Displayed Decay Fits Parameters"=w287:dbl[])  [unwired: 7 in, 1 out]
                n72 = Not(x=w291) -> (.not. x?=w301:bool)
                n73 = Unbundle By Name(w276) -> ("Fit Options.Fit Model"=w275:T2)
                n74 = Build Array (concatenate)(w284, w288) -> (w290:dbl[])
                n75 = case shown="True" w312 {
                  tunnel: [_ w335] -> w313
                  tunnel: w290 -> [_ w334]
                  frame False {
                  }
                  frame True {
                    n76 = Array To Spreadsheet String(array=w334, 3:"%#g" ("format string")) -> (spreadsheet string=w335:string)  [unwired: 1 in]
                  }
                }
                n77 = Build Array (concatenate)(w284, w287) -> (w309:dbl[])
                n78 = call "Tiny Clear Error.vi"("Error In"=w282) -> ("no Error Out"=w314:errorcluster)  [unwired: 8 in]
                n79 = Compound Arithmetic op=AND(w289, w301) -> (w310:bool)
              }
              frame True {
              }
            }
            n80 = call "Send Embedded Progress Bar Update.vi"("Error In"=w250, "Current Iteration i (i or -1: standard or || iteration; 0 or -2: first standard or || iteration)"=-1 ("Current Iteration i (-1: || iteration, -2: first || iteration)"), "Progress Bar Queue in"=w251) -> ("Error Out"=w248:errorcluster, "Progress Bar Queue out"=w249:refnum<queue>)  [unwired: 7 in]
          }
          n81 = Array Size(array=w140) -> (size(s)=w139:i32)
          n82 = Add Array Elements(numeric array=w138) -> (sum=w137:i32)
          n83 = global write "AlliGator Abort.vi" "Abort?"(w167) -> ()
          n84 = Index Array(array=w186) -> (element=w161:T34)  [unwired: 1 in]
          n85 = Equal?(x=w139, y=w137) -> (x = y?=w135:bool)
          n86 = call "XY Graph Add Data to Last Plots.vi"("error in (no error)"=w168, "Plots Data Array"=w170, "XYGraph in"=w169) -> ("error out"=w215:errorcluster)  [unwired: 8 in]
          n87 = call "Send Embedded Progress Bar Update.vi"("Stop Progress Bar (F)"=TRUE, "Error In"=w173, "Progress Bar Queue in"=w174) -> ()  [unwired: 7 in, 2 out]
          n88 = Select(t=w145, s=w132, f=w146) -> (s? t:f=w149:bool)
          n89 = Select(t=w192, s=w132, f=w187) -> (s? t:f=w190:dbl[][])
          n90 = Select(t=w195, s=w132, f=w171) -> (s? t:f=w194:T3[])
          n91 = Select(t=w164, s=w132, f=w166) -> (s? t:f=w165:dbl[][])
          n92 = Select(t=w185, s=w132, f=w161) -> (s? t:f=w184:T34)
          n93 = Select(t=w163, s=w132, f=w140) -> (s? t:f=w162:dbl[])
          n94 = Select(t=w196, s=w132, f=w198) -> (s? t:f=w197:dbl[][])
          n95 = Select(t=w143, s=w132, f=w144) -> (s? t:f=w147:i32)
          n96 = Select(t=w193, s=w132, f=w189) -> (s? t:f=w191:dbl[])
          n97 = Select(t=w136, s=w132, f=w135) -> (s? t:f=w134:bool)
          n98 = Select(t=w141, s=w132, f=w142) -> (s? t:f=w148:i32)
          n99 = Select(t=w160, s=w132, f=w158) -> (s? t:f=w159:T44)
          n100 = Select(t=w157, s=w132, f=w156) -> (s? t:f=w155:cluster{"t Array":dbl[], "I Array":dbl[]})
          n101 = Select(t=w133, s=w132, f=w131) -> (s? t:f=w130:T2)
        }
        frame True {
          n102 = xnode "Error Ring"() -> ("error out"=w350:errorcluster)
        }
      }
      n103 = in-place-cluster #2("Fit Model"=w28, "NLSF Parameters Map X Resolution"=w34, "NLSF Parameters Map Y Resolution"=w33, "Is Full Image Parameters Map"=w42, "Current Dataset Images 1.SGL Sum Image"=w49, "Current Dataset Images 1.SGL Gate Images"=w48, "Current Dataset Images 2.SGL Sum Image"=w67, "Current Dataset Images 2.SGL Gate Images"=w66, "Reference Decay"=w64, "[[Multiple Decays Fit Parameters]]"=w92, "[Decay Fit Parameter Names]"=w76, "IRF Array Time Axis"=w73, "[[IRFs]]"=w72, "Decay Fit Options & Parameters"=w70, "[[Multiple Decays Fit Parameter SDVs]]"=w53, "[Decay Sum]"=w50, "Fit Options: Decay Preprocessing Parameters"=w46, "Fit Options: Reference Decay"=w44, "Is Single-Pixels Parameters Map"=w30) -> (w26:T13)
      n104 = call "AlliGator Get Tabulated Results Header (Decay Fit).vi"("Error In"=w79) -> ("Error Out"=w78:errorcluster, "Tabulated Results Header"=w98:string)  [unwired: 9 in]
      n105 = Build Array (concatenate)(w98, w99) -> (w97:string[])
      n106 = case shown="False" w96 {
        tunnel: w97 -> [w360 _]
        tunnel: [w359 w366] -> w95
        tunnel: w78 -> [w358 w366]
        tunnel: "Choose or enter file path for tabulated fits results:" ("prompt (Choose or enter file path)") -> [w357 _]
        tunnel: w93 -> [w356 _]
        frame False {
          n107 = case shown="True" w356 {
            tunnel: w360 -> [_ w365]
            tunnel: [w361 w364] -> w359
            tunnel: w358 -> [w361 w363]
            tunnel: w357 -> [_ w362]
            frame False {
            }
            frame True {
              n108 = Write to Text File(prompt (Choose or enter file path)=w362, text=w365, error in=w363) -> (error out=w364:errorcluster)  [unwired: 1 in, 2 out]
            }
          }
        }
        frame True {
        }
      }
    }
    n109 = in-place-dvr #1(w26) -> (→"AlliGator Internal Variables DVR":refnum<data-value>)  [unwired: 1 out]
  }
  n110 = call "High Resolution Timing.vi"("relative seconds (NaN)"=w14, "Error In"=w7) -> ("elapsed (relative) seconds"=w13:dbl, "Error Out"=w8:errorcluster)  [unwired: 15 in, 1 out]
  n111 = Array Size(array=w11) -> (size(s)=w10:i32)
  n112 = call "Concatenate String Array.vi"("Max Number of Elements (None: -1)"=8 ("Max Number of Elements (None: 1)"), "Separator (TAB)"=", ", "String Array"=w11) -> ("Formatted String"=w12:string)  [unwired: 8 in]
  n113 = call "Current Date & Time String (High Precision).vi"("Error In"=w8) -> ("on <Date> at <Time>"=w1:string)  [unwired: 7 in, 3 out]
  n114 = Format Into String(format string="All ROIs Decay Fit (%d):\n%scompleted %s\nCPU: %#g s\n", error in=w8, w10, w12, w1, w13) -> (resulting string=→"Message":string, error out=→"error out":errorcluster)  [unwired: 1 in]
